vi "Simple Execute.vi"(7 "Return Report? (F)":bool, 8 "error in (no error)":errorcluster, 9 "Parameters (None)":T2, 10 "Entry Point / Sequence":string(combo), 11 "Session Handle in":T3) -> (0 "error out":errorcluster, 1 "Report":T1, 2 "Status":string, 3 "Session Handle out":T3)   [LabVIEW 2020, in "TSS.lvlib" / "SequenceFile.lvclass"]
uses:
  SequenceFile.lvclass
  Typedefs/Session Handle.ctl
  VariableContainer/Typedefs/Session Handle.ctl
  VariableContainer/VariableContainer.lvclass
  Report/Typedefs/Session Handle.ctl
  Report/Report.lvclass
  Execution/Execution Options.ctl
  Get Engine.vi
  Execution/Set Sequence File.vi
  Execution/Set Entry Sequence.vi
  Execution/Set Parameters.vi
  Execution/Get Result Status.vi
  Engine/Engine.lvclass
  Execution/Execution.lvclass
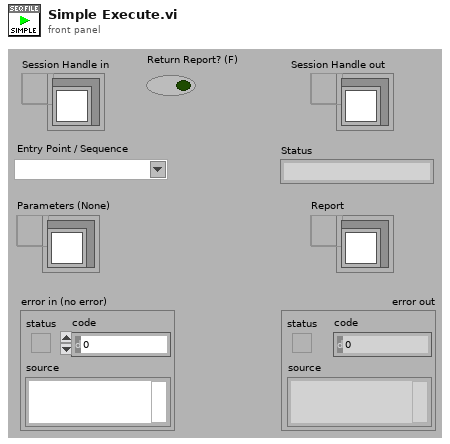
[diagram p1: front panel]
types:
  T1 = typedef "TSS.lvlib/Report.lvclass/Session Handle.ctl" = refnum<data-value>
  T2 = typedef "TSS.lvlib/VariableContainer.lvclass/Session Handle.ctl" = refnum<data-value>
  T3 = typedef "TSS.lvlib/SequenceFile.lvclass/Session Handle.ctl" = refnum<data-value>
  T4 = typedef "TSS.lvlib/Execution.lvclass/Execution Options.ctl" = cluster{"Use Default Model":bool, "Release Related Sessions":bool}
  T5 = typedef "TSS.lvlib/Engine.lvclass/Session Handle.ctl" = refnum<data-value>
  T6 = typedef "TSS.lvlib/Execution.lvclass/Session Handle.ctl" = refnum<data-value>
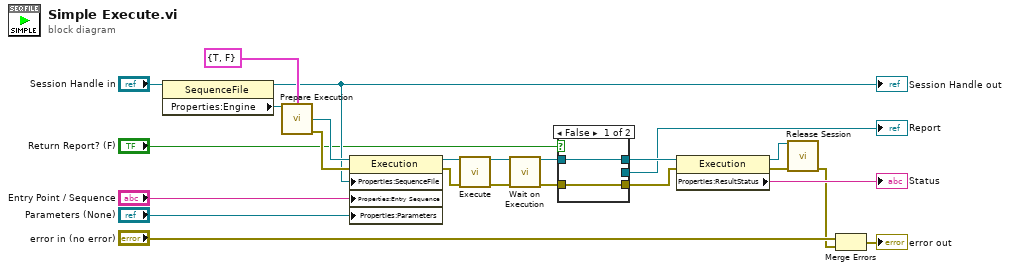
[diagram p0: block diagram]
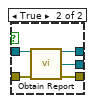
[diagram p2: hidden frame]
diagram:
  n1 = property class="SequenceFile"(reference="Session Handle in") -> (reference out=w2:T3, "Properties:Engine"=w22:T5)  [unwired: 1 in, 1 out]
  "Session Handle out" <- w2
  n2 = call "Prepare Execution.vi"("Session Handle in"=w22, "Options (Default)"=T4 {"Use Default Model"=TRUE, "Release Related Sessions"=FALSE}) -> ("Execution"=w21:T6, "error out"=w20:errorcluster)  [unwired: 11 in, 1 out]
  n3 = property class="Execution"(reference=w21, error in=w20, "Properties:SequenceFile"=w2, "Properties:Entry Sequence"="Entry Point / Sequence", "Properties:Parameters"="Parameters (None)") -> (reference out=w17:T6, error out=w16:errorcluster)
  n4 = call "Execute.vi"("Session Handle in"=w17, "error in (no error)"=w16) -> ("Session Handle out"=w15:T6, "error out"=w14:errorcluster)  [unwired: 12 in]
  n5 = call "Wait on Execution.vi"("Session Handle in"=w15, "error in (no error)"=w14) -> ("Session Handle out"=w13:T6, "error out"=w12:errorcluster)  [unwired: 11 in, 1 out]
  n6 = case shown="False" "Return Report? (F)" {
    tunnel: w13 -> [w26 w31]
    tunnel: w12 -> [w25 w30]
    tunnel: [w26 w29] -> w11
    tunnel: [w25 w28] -> w10
    tunnel: [_ w27] -> w9
    frame False {
    }
    frame True {
      n7 = call "Obtain Report.vi"("Session Handle in"=w31, "error in (no error)"=w30) -> ("Session Handle out"=w29:T6, "Report"=w27:T1, "error out"=w28:errorcluster)  [unwired: 11 in]
    }
  }
  "Report" <- w9
  n8 = property class="Execution"(reference=w11, error in=w10) -> (reference out=w5:T6, error out=w6:errorcluster, "Properties:ResultStatus"=→"Status":string)
  n9 = call "Release Session.vi"("Session Handle"=w5, "error in (no error)"=w6) -> ("error out"=w3:errorcluster)  [unwired: 13 in]
  n10 = Merge Errors("error in (no error)", w3) -> (→"error out":errorcluster)
